vi "Read Measurement (Voltage Time).vi"(0 "VISA resource name":refnum<visa-resource-name>, 5 "Channel (1: Channel 1)":u16(ring) items=["Channel 1", "Channel 2", "Channel 3", "Channel 4", "Function 1", "Function 2", "Function 3", "Function 4", "Memory 1", "Memory 2", "Memory 3", "Memory 4"], 7 "Delay (500e-3)":dbl format="%#_6f", 9 "Maximum Time (10000ms)":u32, 11 "error in (no error)":errorcluster) -> (4 "VISA resource name out":refnum<visa-resource-name>, 6 "Time Voltage (v)":dbl, 15 "error out":errorcluster)   [LabVIEW 2009, in "Agilent 8000 Series.lvlib"]
doc: "Returns the voltage at a specified time. The specified time must be on screen and referenced to the trigger event. When an FFT function is the specified source, the amplitude at the specified frequency is measured, the returned value is the vertical value at the horizontal setting passed in the delay parameter. \n\nThis VI initiates an acquisition on the channel that the end-user defined. It then waits for the acquisition to complete, obtains a waveform measurement on the channel the end-user specifies, and returns the measurement value."
uses:
  Agilent 8000 Series.lvlib
  Low Level/Fetch Measurement (Voltage Time).vi
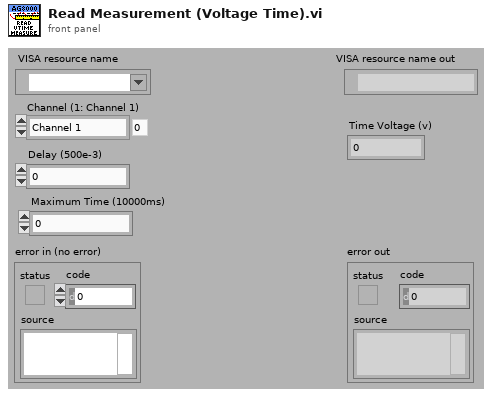
[diagram p1: front panel]
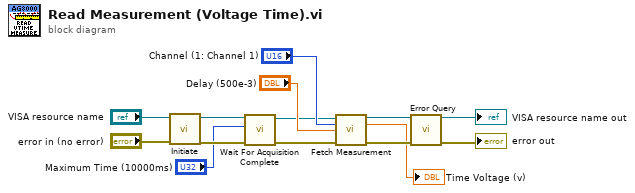
[diagram p0: block diagram]
diagram:
  n1 = call "Initiate.vi"("error in (no error)"="error in (no error)", "VISA resource name"="VISA resource name") -> ("error out"=w2:errorcluster, "VISA resource name out"=w5:refnum<visa-resource-name>)  [unwired: 8 in]
  n2 = call "Wait For Acquisition Complete.vi"("error in (no error)"=w2, "Maximum Time (10000ms)"="Maximum Time (10000ms)", "VISA resource name"=w5) -> ("error out"=w3:errorcluster, "VISA resource name out"=w4:refnum<visa-resource-name>)  [unwired: 7 in]
  n3 = call-poly "Fetch Measurement.vi"("VISA resource name"=w4, "Channel (1: Channel 1)"="Channel (1: Channel 1)", "Delay (500e-3)"="Delay (500e-3)", "error in (no error)"=w3) -> ("VISA resource name out"=w10:refnum<visa-resource-name>, "Time Voltage (s)"=→"Time Voltage (v)":dbl, "error out"=w9:errorcluster)  [unwired: 9 in]
  n4 = call "Error Query.vi"("error in (no error)"=w9, "VISA resource name"=w10) -> ("error out"=→"error out":errorcluster, "VISA resource name out"=→"VISA resource name out":refnum<visa-resource-name>)  [unwired: 6 in, 2 out]
